vi "fruit_detectorr(1).vi"() -> ()   [LabVIEW 2017]
uses:
  <vilib>/Instr/_visa.llb/VISA Configure Serial Port (Instr).vi
  <vilib>/addons/Fuzzy Logic/FL Fuzzy Controller (MISO).vi
  <vilib>/addons/Fuzzy Logic/NI_Fuzzy_Logic_API.lvlib
panel:
  out "element":u32
  in  "stop":bool
  in  "stop 3":bool
  in  "byte count":u32
  out "read buffer":string
  in  "VISA resource":refnum<visa-resource-name>
  in  "Image Type":T1 items=["Grayscale (U8)", "Grayscale (I16)", "Grayscale (SGL)", "Complex (CSG)", "RGB (U32)", "HSL (U32)", "RGB (U64)", "Grayscale (U16)"]
  in  "File Path":path
  out "Image":T2(plugin-control)
  out "Numeric":dbl
  out "String":string="coconut"
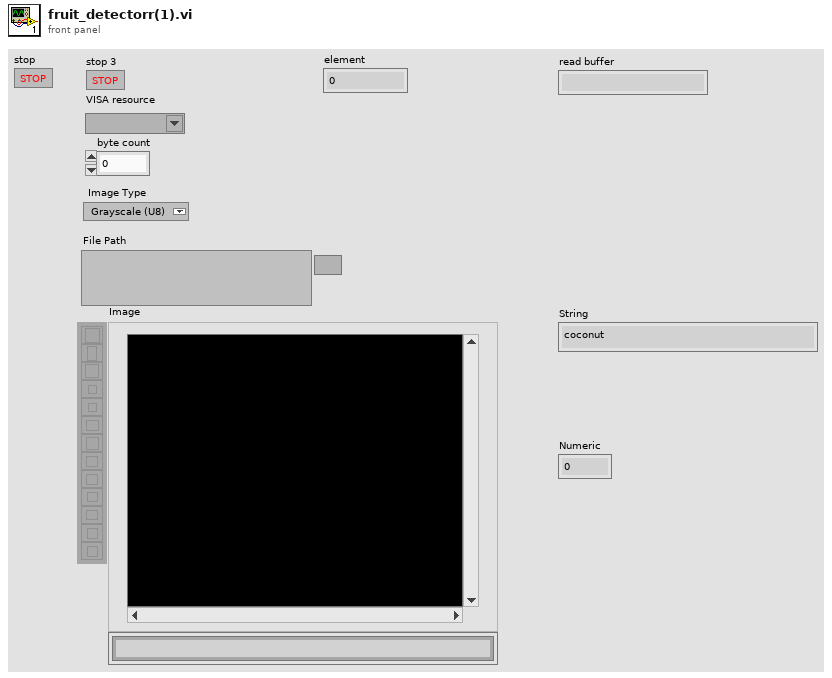
[diagram p1: front panel]
types:
  T1 = typedef "Image Type" = u32
  T2 = typedef "IMAQ Image.ctl" = refnum<image>
  T3 = typedef "NI_Fuzzy_Logic_API.lvlib/FL System.ctl" = cluster{"input variables":T4[], "output variables":T4[], "rules":T7[], "defuzzification method":T13, "description":string, "user MF interpolating polynomials":T14[]}
  T4 = typedef "NI_Fuzzy_Logic_API.lvlib/FL Variable.ctl" = cluster{"name":string, "range":dbl[], "MFs":T5[]}
  T5 = typedef "NI_Fuzzy_Logic_API.lvlib/FL Membership Function.ctl" = cluster{"name":string, "shape":T6, "points":dbl[], "color":u32, "user-defined shape index":i32}
  T6 = typedef "NI_Fuzzy_Logic_API.lvlib/FL Membership Function Shape.ctl" = u16
  T7 = typedef "NI_Fuzzy_Logic_API.lvlib/FL Rule.ctl" = cluster{"antecedents":T8[], "antecedent connective":T10, "consequents":T11[], "consequent implication":T12, "degree of support":dbl}
  T8 = typedef "NI_Fuzzy_Logic_API.lvlib/FL Antecedent.ctl" = cluster{"Var Index":i32, "MF Index":i32, "Cond":T9}
  T9 = typedef "NI_Fuzzy_Logic_API.lvlib/FL Modifier.ctl" = u16
  T10 = typedef "NI_Fuzzy_Logic_API.lvlib/FL Antecedent Connective.ctl" = u16
  T11 = typedef "NI_Fuzzy_Logic_API.lvlib/FL Consequent.ctl" = cluster{"Var Index":i32, "MF Index":i32, "Cond":T9}
  T12 = typedef "NI_Fuzzy_Logic_API.lvlib/FL Consequent Implication.ctl" = u16
  T13 = typedef "NI_Fuzzy_Logic_API.lvlib/FL Defuzzification.ctl" = u16
  T14 = typedef "NI_Fuzzy_Logic_API.lvlib/FL Interpolating polynomials.ctl" = cluster{"X":dbl[], "Y":dbl[], "Y(x) coeff":dbl[][], "X(y) coeff":dbl[][], "Area(y) coeff":dbl[][], "coa_x(y) coeff":dbl[][]}
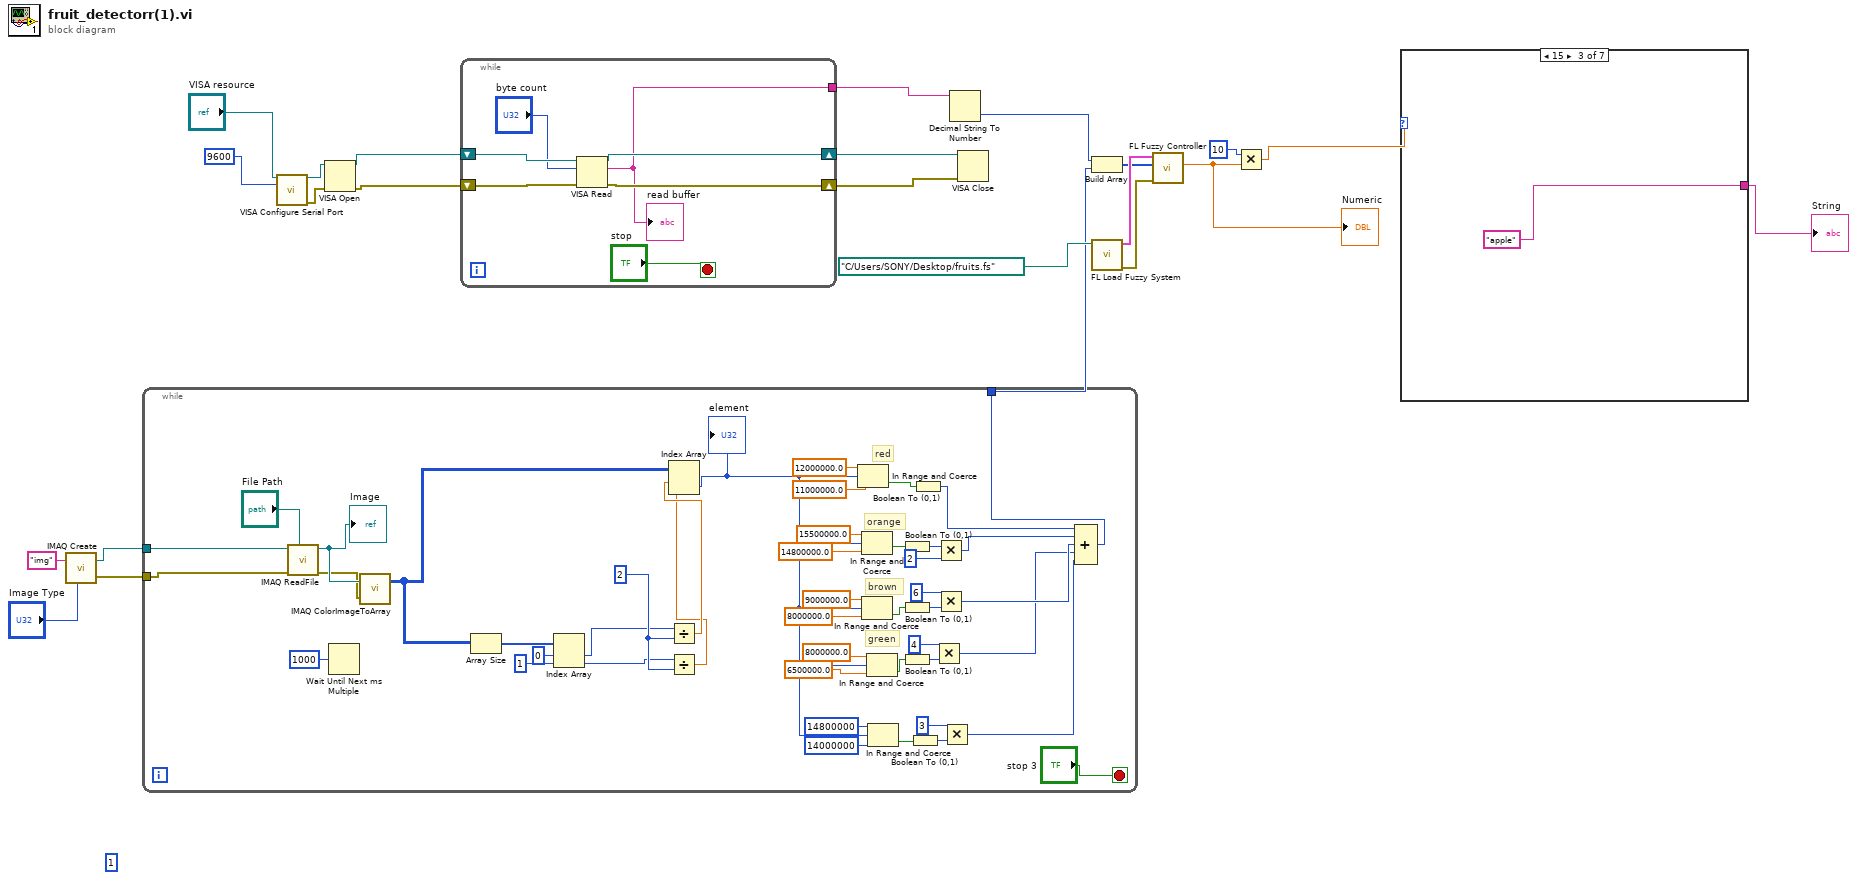
[diagram p0: block diagram]
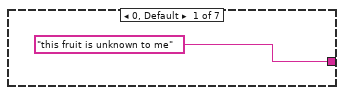
[diagram p2: hidden frame]
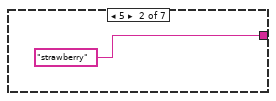
[diagram p3: hidden frame]
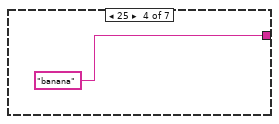
[diagram p4: hidden frame]
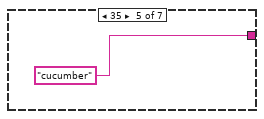
[diagram p5: hidden frame]
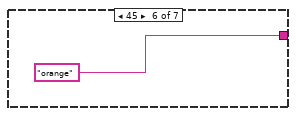
[diagram p6: hidden frame]
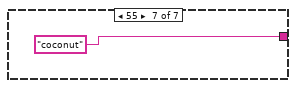
[diagram p7: hidden frame]
diagram:
  (unwired) 1
  n1 = call "IMAQ Create"("Image Name"="img", "Image Type"="Image Type") -> ("New Image"=w5:T2, "error out"=w4:errorcluster)  [unwired: 3 in]
  n2 = while {
    tunnel: [w69] -> w16
    tunnel: w5 -> [w28]
    tunnel: w4 -> [w27]
    stop <- "stop 3" stop-if-true
    w65 = 2
    # "orange"
    # "brown"
    # "green"
    # "red"
    n3 = call "IMAQ ReadFile"("File Path"="File Path", "error in (no error)"=w27, "Image"=w28) -> ("error out"=w25:errorcluster, "Image Out"=w30:T2)  [unwired: 4 in, 3 out]
    "Image" <- w30
    n4 = Wait Until Next ms Multiple(millisecond multiple=u32 1000) -> ()  [unwired: 1 out]
    n5 = call "IMAQ ColorImageToArray"("Image"=w30, "error in (no error)"=w25) -> ("Image Pixels (U32)"=w62:u32[][])  [unwired: 2 in, 2 out]
    n6 = Array Size(array=w62) -> (size(s)=w68:i32[])
    n7 = Index Array(array=w68, index #1=0 ("index"), index #2=1 ("index")) -> (element #1=w64:i32, element #2=w63:i32)
    n8 = Divide(x=w64, y=w65) -> (x/y=w61:dbl)
    n9 = Divide(x=w63, y=w65) -> (x/y=w60:dbl)
    n10 = Index Array(array=w62, index (row)=w61, index (col)=w60) -> (element=w38:u32)
    "element" <- w38
    n11 = In Range and Coerce(upper limit=12000000.0, x=w38, lower limit=11000000.0) -> (In Range?=w45:bool)  [unwired: 1 out]
    n12 = In Range and Coerce(upper limit=15500000.0, x=w38, lower limit=14800000.0) -> (In Range?=w47:bool)  [unwired: 1 out]
    n13 = In Range and Coerce(upper limit=9000000.0, x=w38, lower limit=8000000.0) -> (In Range?=w46:bool)  [unwired: 1 out]
    n14 = In Range and Coerce(upper limit=8000000.0, x=w38, lower limit=6500000.0) -> (In Range?=w49:bool)  [unwired: 1 out]
    n15 = In Range and Coerce(upper limit=u32 14800000, x=w38, lower limit=u32 14000000) -> (In Range?=w33:bool)  [unwired: 1 out]
    n16 = Boolean To (0,1)(Boolean=w47) -> (0, 1=w51:i16)
    n17 = Boolean To (0,1)(Boolean=w46) -> (0, 1=w50:i16)
    n18 = Boolean To (0,1)(Boolean=w49) -> (0, 1=w48:i16)
    n19 = Boolean To (0,1)(Boolean=w33) -> (0, 1=w34:i16)
    n20 = Boolean To (0,1)(Boolean=w45) -> (0, 1=w44:i16)
    n21 = Multiply(x=i16 4, y=w48) -> (x*y=w24:i16)
    n22 = Multiply(x=w51, y=i16 2) -> (x*y=w40:i16)
    n23 = Multiply(x=i16 6, y=w50) -> (x*y=w39:i16)
    n24 = Multiply(x=i16 3, y=w34) -> (x*y=w32:i16)
    n25 = Compound Arithmetic op=ADD(w44, w40, w39, w24, w32) -> (w69:i16)
  }
  n26 = call-poly "VISA Configure Serial Port"("VISA resource name"="VISA resource", "baud rate (9600)"=u32 9600 ("Baud Rate (115200)")) -> ("VISA resource name out"=w9:refnum<visa-resource-name>, "error out"=w15:errorcluster)  [unwired: 12 in]
  n27 = VISA Open(error in (no error)=w15, VISA resource name=w9) -> (VISA resource name=w12:refnum<visa-resource-name>, error out=w11:errorcluster)  [unwired: 3 in]
  n28 = while {
    shift-right: [w76] -> w14
    shift-left: w12 -> [w74]
    shift-right: [w75] -> w13
    shift-left: w11 -> [w73]
    tunnel: [w70] -> w2
    stop <- "stop" stop-if-true
    n29 = VISA Read(VISA resource name=w74, byte count="byte count", error in (no error)=w73) -> (VISA resource name out=w76:refnum<visa-resource-name>, read buffer=w70:string, error out=w75:errorcluster)  [unwired: 1 out]
    "read buffer" <- w70
  }
  n30 = Decimal String To Number(string=w2) -> (number=w1:i32)  [unwired: 2 in, 1 out]
  n31 = VISA Close(VISA resource name=w14, error in (no error)=w13) -> ()  [unwired: 1 out]
  n32 = Build Array(w1, w16) -> (w3:i32[])
  n33 = call <vilib>:"FL Load Fuzzy System.vi"("file path"=path "C:/Users/SONY/Desktop/fruits.fs") -> ("error out"=w22:errorcluster, "fuzzy system out"=w23:T3)  [unwired: 9 in]
  n34 = call-poly <vilib>:"FL Fuzzy Controller.vi"("error in (no error)"=w22, "input values"=w3, "fuzzy system in"=w23) -> ("output value"=w19:dbl)  [unwired: 4 in, 4 out]
  "Numeric" <- w19
  n35 = Multiply(x=10, y=w19) -> (x*y=w18:dbl)
  n36 = case shown="15" w18 {
    tunnel: ["this fruit is unknown to me" "strawberry" "apple" "banana" "cucumber" "orange" "coconut"] -> w17
    frame 0, Default {
    }
    frame 5 {
    }
    frame 15 {
    }
    frame 25 {
    }
    frame 35 {
    }
    frame 45 {
    }
    frame 55 {
    }
  }
  "String" <- w17
